vi "Springboard Demo - place and adjust arrows.vi"() -> ()   [LabVIEW 2025]
uses:
  <vilib>/Utility/miscctls.llb/LVPositionTypeDef.ctl
  <vilib>/Utility/miscctls.llb/LVBoundsTypeDef.ctl
  Arrow Direction.ctl
panel:
  in  "Arrow Direction":T1
  in  "stop":bool
  in  "Size":T2 {"Width" scale=5.0..100.0; "Height" scale=5.0..100.0}
  in  "Position":T3 {"Left" scale=-100.0..100.0; "Top" scale=-100.0..100.0}
  in  "ACTION":bool
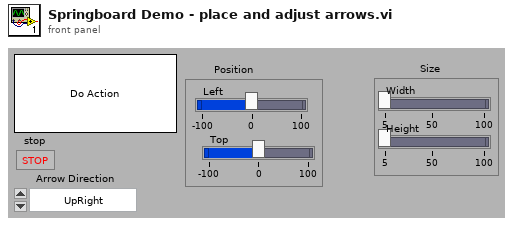
[diagram p1: front panel]
types:
  T1 = typedef "Arrow Direction.ctl" = enum16{"UpRight", "UpLeft", "DownLeft", "DownRight"}
  T2 = typedef "LVBoundsTypeDef.ctl" = cluster{"Width":u32, "Height":u32}
  T3 = typedef "LVPositionTypeDef.ctl" = cluster{"Left":i32, "Top":i32}
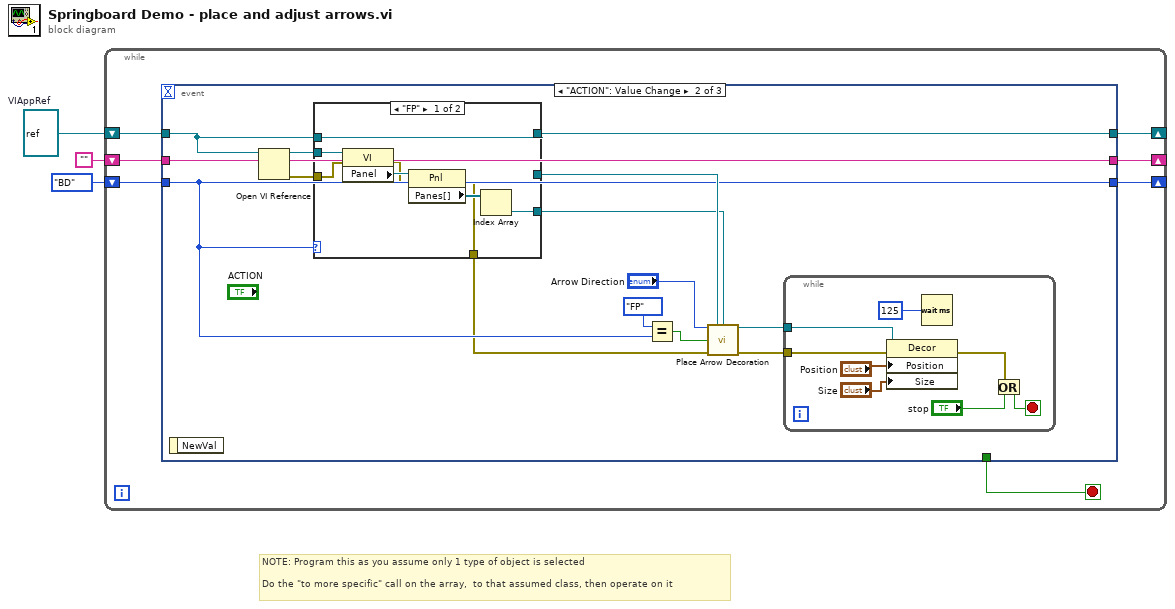
[diagram p0: block diagram]
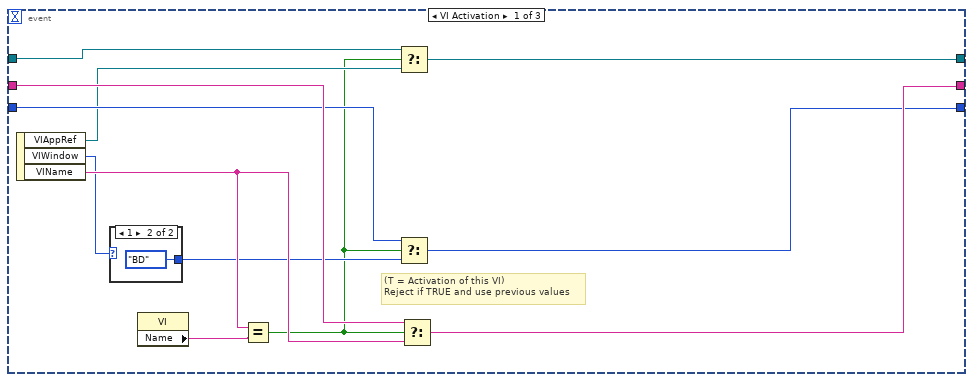
[diagram p2: hidden frame]
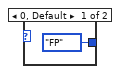
[diagram p3: hidden frame]
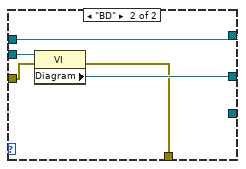
[diagram p4: hidden frame]
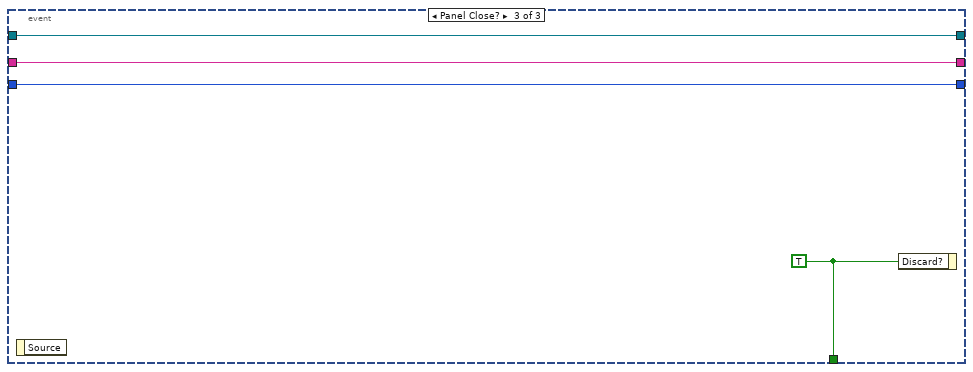
[diagram p5: hidden frame]
diagram:
  w1 = refnum<vi> refnum  # VIAppRef
  # "NOTE: Program this as you assume only 1 type of object is selected\n\nDo the \"to more specific\" call on the array,  to that assumed class, then operate on it"
  n1 = while {
    shift-right: [w10] -> _
    shift-left: "" -> [w9]
    shift-right: [w7] -> _
    shift-left: enum16{"FP", "BD"}."BD" -> [w6]
    shift-right: [w5] -> _
    shift-left: w1 -> [w4]
    stop <- w8 stop-if-true
    n2 = event shown="[1] \"ACTION\": Value Change" {
      selector: _ -> [_ _ _]
      dyn-events: _ -> [_ _ _]
      timeout: _ -> [_ _ _]
      tunnel: [w19 w35 w61] -> w10
      tunnel: w9 -> [w22 w35 w61]
      tunnel: [_ _ w63] -> w8
      tunnel: [w17 w28 w62] -> w7
      tunnel: w6 -> [w18 w28 w62]
      tunnel: [w13 w37 w60] -> w5
      tunnel: w4 -> [w12 w36 w60]
      event VI Activation {
        # "(T = Activation of this VI)\nReject if TRUE and use previous values"
        n3 = event-data() -> ("VIAppRef"=w14:refnum<vi>, "VIWindow"=w16:i32, "VIName"=w20:string)  [unwired: 1 out]
        n4 = case shown="1" w16 {
          tunnel: [enum16{"FP", "BD"}."FP" enum16{"FP", "BD"}."BD"] -> w15
          frame 0, Default {
          }
          frame 1 {
          }
        }
        n5 = property class="VI"() -> ("Name"=w21:string)  [unwired: 2 in, 2 out]
        n6 = Equal?(x=w20, y=w21) -> (x = y?=w11:bool)
        n7 = Select(t=w12, s=w11, f=w14) -> (s? t:f=w13:refnum<vi>)
        n8 = Select(t=w18, s=w11, f=w15) -> (s? t:f=w17:enum16{"FP", "BD"})
        n9 = Select(t=w22, s=w11, f=w20) -> (s? t:f=w19:string)
      }
      event "ACTION": Value Change {
        n10 = event-data() -> ()  [unwired: 2 out]
        n11 = Open VI Reference(application reference (local)=w36, vi path=w35) -> (vi reference=w38:refnum<vi>, error out=w26:errorcluster)  [unwired: 2 in, 2 out]
        n12 = case shown="\"FP\"" w28 {
          tunnel: w38 -> [w54 w59]
          tunnel: [w52 w58] -> w37
          tunnel: w36 -> [w52 w58]
          tunnel: [_ w57] -> w33
          tunnel: [w50 _] -> w32
          tunnel: w26 -> [w49 w56]
          tunnel: [w47 w55] -> w25
          frame "FP" {
            n13 = property class="VI"(reference=w54, error in=w49) -> (error out=w48:errorcluster, "Panel"=w53:refnum<vi>)  [unwired: 1 out]
            n14 = property class="Pnl"(reference=w53, error in=w48) -> (error out=w47:errorcluster, "Panes[]"=w51:refnum<vi>[])  [unwired: 1 out]
            n15 = Index Array(array=w51) -> (element=w50:refnum<vi>)  [unwired: 1 in]
          }
          frame "BD" {
            n16 = property class="VI"(reference=w59, error in=w56) -> (error out=w55:errorcluster, "Diagram"=w57:refnum<vi>)  [unwired: 1 out]
          }
        }
        n17 = Equal?(x=enum16{"FP", "BD"}."FP", y=w28) -> (x = y?=w27:bool)
        n18 = call "Place Arrow Decoration.vi"("Arrow Direction"="Arrow Direction", "Diagram"=w33, "Pane Refnum"=w32, "FP? (T)"=w27, "error in"=w25) -> ("Decor Refnum"=w31:refnum<vi>, "error out"=w30:errorcluster)  [unwired: 9 in]
        n19 = while {
          tunnel: w31 -> [w43]
          tunnel: w30 -> [w42]
          stop <- w39 stop-if-true
          n20 = property class="Decor"(reference=w43, error in=w42, "Position"="Position", "Size"="Size") -> (error out=w41:errorcluster)  [unwired: 1 out]
          n21 = Wait (ms)(milliseconds to wait=u32 125) -> ()  [unwired: 1 out]
          n22 = Or(x="stop", y=w41) -> (x .or. y?=w39:bool)
        }
      }
      event Panel Close? {
        w63 = TRUE ("Discard?")
        n23 = event-data() -> ()  [unwired: 2 out]
        n24 = event-data("Discard?"=w63) -> ()  [unwired: 1 in, 1 out]
      }
    }
  }
